vi "FPGA-test001.vi"() -> ()   [LabVIEW 2019]
uses:
  Labview/smallmom-3 FPGA test/FPGA-test/Sub VIs/Utilities/Start Boolean.ctl
  <vilib>/Platform/TimedLoop/XDataNode/timing_clust.ctl
  <vilib>/Platform/TimedLoop/XDataNode/nitl_modes.ctl
  <vilib>/Platform/TimedLoop/XDataNode/wakeup.ctl
  <vilib>/rvi/Emulation/niFpgaGetClockAttributes.vi
  <vilib>/rvi/Emulation/niFpgaSctlEmulationGetInTimedLoop.vi
  <vilib>/rvi/Emulation/niFpgaEmulationReportErrorSimple.vi
  <vilib>/rvi/eio/common/nirviEmuTemplateMethod_errors.vi
  <vilib>/rvi/Emulation/niFpgaCriticalErrorInLSC.vi
  <vilib>/eio/EIONode/EIONode.xnode
  <vilib>/platform/TimedLoop/XDataNode/XDataNode.xnode
  <vilib>/Platform/TimedLoop/XDataNode/XDNodeRunTimeDep.lvlib
panel:
  in  "Servo4.period (20Mhz)":u32=60606
  in  "Servo3.period (20Mhz)":u32=60606
  in  "Servo2.period (20Mhz)":u32=60606
  in  "Servo1.period (20Mhz)":u32=60606
  in  "Basic.2 IO Write":u8
  in  "Basic.2 IO DIR":u8
  out "Basic.2 IO Read":u8
  in  "Servo4.pulse(0.05us)":u32
  out "us4.distance":i32
  out "us3.distance":i32
  out "us2.distance":i32
  out "us1.distance":i32
  in  "us4.timeout(us)":i32
  in  "us3.timeout(us)":i32
  in  "us2.timeout(us)":i32
  in  "us1.timeout(us)":i32
  in  "Ultrasonic.IO.Enable":u8 format="%.0b"
  in  "I2C.A.GO":T1
  in  "I2C.A.CNFG":u8=1 format="%08b"
  out "I2C.A.STAT":u8 format="%08b"
  in  "I2C.A.CNTL":u8 format="%08b"
  in  "I2C.A.CNTR":u8=213
  in  "I2C.A.ADDR":u8 format="%08b"
  out "I2C.A.DATI":u8
  in  "I2C.A.DATO":u8
  in  "Ultrasonic.IO.Write":u8
  in  "Ultrasonic.io.DIR":u8
  out "Ultrasonic.io.Read":u8
  out "Basic IO Read":u8
  in  "Basic IO DIR":u8
  in  "Basic IO Write":u8
  out "IR 8":u16
  out "IR 7":u16
  out "IR 6":u16
  out "IR 5":u16
  out "IR 4":u16
  out "IR 3":u16
  out "IR 2":u16
  out "IR 1":u16
  in  "Servo3.pulse(0.05us)":u32
  in  "Servo2.pulse(0.05us)":u32
  in  "Servo1.pulse(0.05us)":u32
  in  "Motor3.encoder_Reset":bool
  out "Motor3.encoder":i32
  in  "Motor3.speed":i64
  in  "Motor3.periode":i64
  in  "Motor3.enable_divider":bool
  in  "Motor3.divider":fxp<+,4,4>
  in  "Motor3.brake":bool
  in  "Motor4.encoder_Reset":bool
  out "Motor4.encoder":i32
  in  "Motor4.speed":i64
  in  "Motor4.periode":i64
  in  "Motor4.enable_divider":bool
  in  "Motor4.divider":fxp<+,4,4>
  in  "Motor4.brake":bool
  in  "Motor2.encoder_Reset":bool
  out "Motor2.encoder":i32
  in  "Motor2.speed":i64
  in  "Motor2.periode":i64
  in  "Motor2.enable_divider":bool
  in  "Motor2.divider":fxp<+,4,4>
  in  "Motor2.brake":bool
  in  "Motor1.brake":bool
  in  "Motor1.divider":fxp<+,4,4>
  in  "Motor1.enable_divider":bool
  in  "Motor1.periode":i64
  in  "Motor1.speed":i64
  out "Motor1.encoder":i32
  in  "Motor1.encoder_Reset":bool
  out "OnBoard.BUTTON":bool
  in  "OnBoard.LED[3:0]":fxp<+,4,4> format="%.0b"
  # "Motor1"
  # "Motor2"
  # "Motor3"
  # "Motor4"
  # "Servo"
  # "IR Sensor"
  # "Basic IO"
  # "Ultrasonic IO"
  # "I2C"
  # "OnBoard"
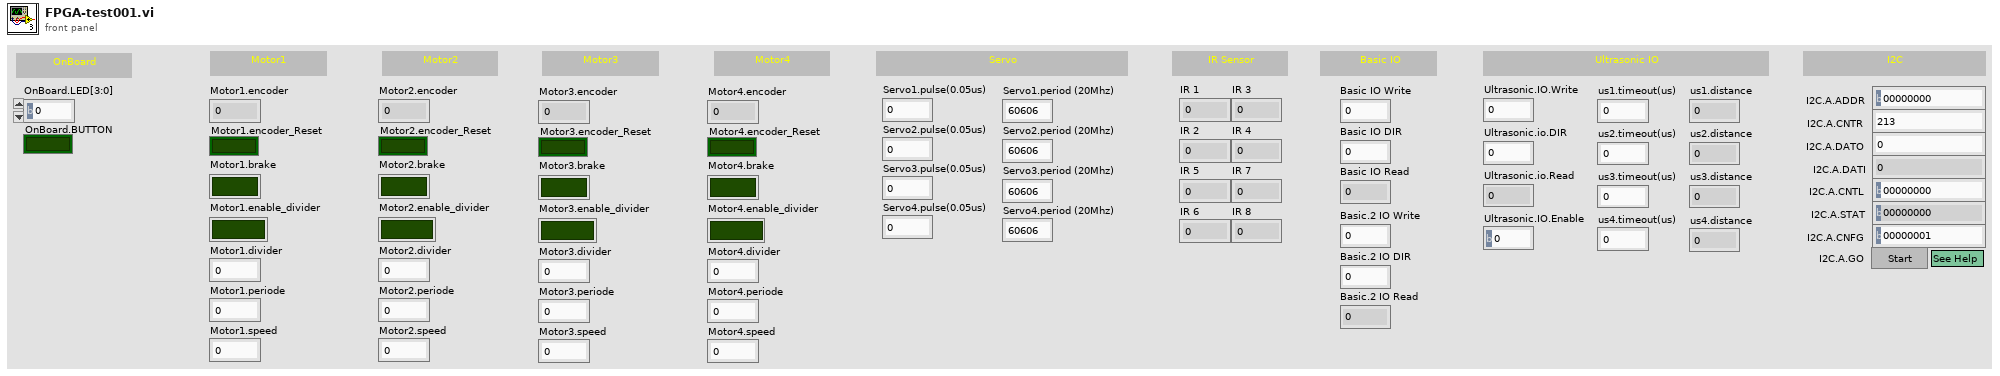
[diagram p1: front panel]
types:
  T1 = typedef "Start Boolean.ctl" = bool
  T2 = typedef "XDNodeRunTimeDep.lvlib/timing_clust.ctl" = cluster{"Expected End [f-1]":u64, "Actual End [f-1]":u64, "Finished Late? [f-1]":bool, "Expected End [i-1]":u64, "Actual End [i-1]":u64, "Finished Late? [i-1]":bool, "Expected Start [i]":u64, "Actual Start [i]":u64, "Expected Start [f]":u64, "Actual Start [f]":u64, "Source Name":string, "Structure Name":string, "Period":i64, "Deadline":i64, "Offset":i64, "Start":i64, "Priority":i32, "Timeout":i32, "Mode":T3, "Wakeup Reason":T4, "Error":errorcluster, "Source Type":string, "Secondary Source Type":string, "Global End Time":u64, "Global Start Time":u64, "Frame Duration":u64, "Iteration Duration":u64, "Assigned CPU":i32, "I/O Scan Engine Mode":u32}
  T3 = typedef "XDNodeRunTimeDep.lvlib/nitl_modes.ctl" = enum32{"No Change", "Process missed periods, maintain original phase", "Discard missed periods, maintain original phase", "Process missed periods, ignore original phase", "Discard missed periods, ignore original phase"}
  T4 = typedef "XDNodeRunTimeDep.lvlib/wakeup.ctl" = enum32{"Normal", "Aborted", "Asynchronous wakeup", "Timing source error", "Timed loop error", "Timeout"}
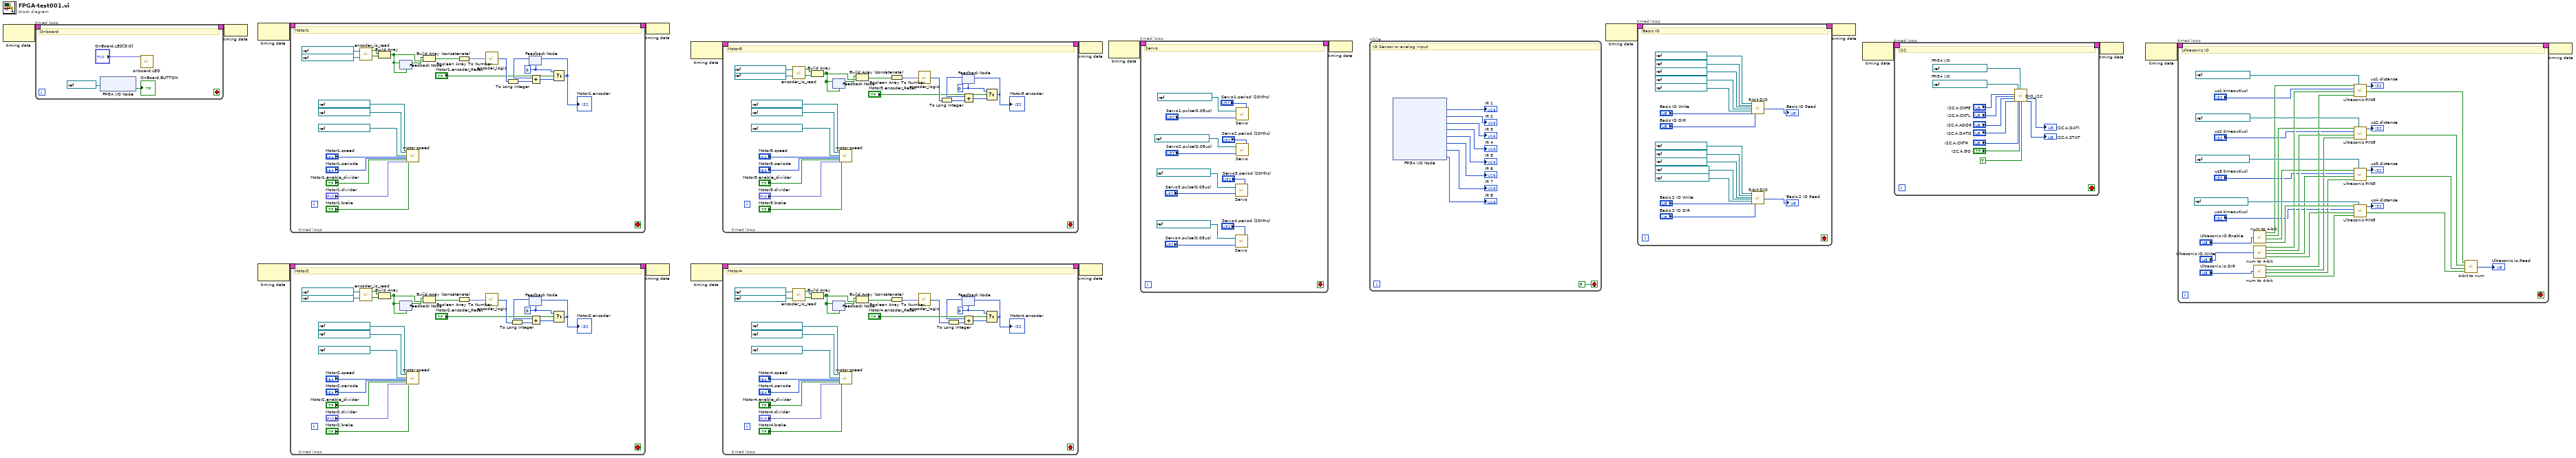
[diagram p0: block diagram]
diagram:
  n1 = node-c288() -> (w18:T2)  [unwired: 1 in]
  n2 = timed-loop "Timed Loop" {
    timing: w18 -> [_]
    timing-out: [_] -> w17
    stop <- _ stop-if-true
    # "Onboard"
    n3 = xnode "FPGA I/O Node"("FPGA I/O In"=refnum<k21> "Button0") -> ("I/O Item"=→"OnBoard.BUTTON":bool)  [unwired: 1 out]
    n4 = call "onboard.LED.vi"("OnBoard.LED[3:0]"="OnBoard.LED[3:0]") -> ()  [unwired: 11 in]
  }
  n5 = node-c288(w17) -> ()
  n6 = node-c288() -> (w16:T2)  [unwired: 1 in]
  n7 = node-c288() -> (w14:T2)  [unwired: 1 in]
  n8 = timed-loop "Timed Loop" {
    timing: w16 -> [_]
    timing-out: [_] -> w15
    stop <- _ stop-if-true
    w37 = 0
    # "Motor1"
    n9 = call "encoder_io_read.vi"("PhaseB"=refnum<k21> "ConnectorA/DIO3", "PhaseA"=refnum<k21> "ConnectorA/DIO2") -> ("PhaseB"=w44:bool, "PhaseA"=w45:bool)
    n10 = Build Array(w45, w44) -> (w42:bool[])
    n11 = feedback-in #1(w42) -> ()
    n12 = feedback #1(w42) -> (w43:bool[])
    n13 = call "motor speed.vi"("IN_A"=refnum<k21> "ConnectorA/DIO0" ("PhaseA"), "IN_B"=refnum<k21> "ConnectorA/DIO1" ("PhaseB"), "PWM"=refnum<k21> "ConnectorA/DIO4" ("PhaseB"), "speed"="Motor1.speed", "periode"="Motor1.periode", "enable divider"="Motor1.enable_divider", "divider"="Motor1.divider", "brake"="Motor1.brake") -> ()  [unwired: 20 in]
    n14 = Build Array (concatenate)(w43, w42) -> (w33:bool[])
    n15 = Boolean Array To Number(Boolean array=w33) -> (number=w41:fxp<+,4,4>)
    n16 = call "encoder_logic.vi"("encoder"=w41) -> ("out"=w39:i16)
    n17 = To Long Integer(number=w39) -> (32bit integer=w24:i32)
    n18 = feedback #2(w37) -> (w40:i32)
    n19 = Add(x=w40, y=w24) -> (x+y=w36:i32)
    n20 = Select(t=w37, s="Motor1.encoder_Reset", f=w36) -> (s? t:f=w35:i32)
    "Motor1.encoder" <- w35
    n21 = feedback-in #2(w35) -> ()
  }
  n22 = timed-loop "Timed Loop" {
    timing: w14 -> [_]
    timing-out: [_] -> w13
    stop <- _ stop-if-true
    w62 = 0
    # "Motor2"
    n23 = call "encoder_io_read.vi"("PhaseB"=refnum<k21> "ConnectorA/DIO8", "PhaseA"=refnum<k21> "ConnectorA/DIO7") -> ("PhaseB"=w69:bool, "PhaseA"=w70:bool)
    n24 = Build Array(w70, w69) -> (w67:bool[])
    n25 = feedback-in #3(w67) -> ()
    n26 = feedback #3(w67) -> (w68:bool[])
    n27 = call "motor speed.vi"("IN_A"=refnum<k21> "ConnectorA/DIO5" ("PhaseA"), "IN_B"=refnum<k21> "ConnectorA/DIO6" ("PhaseB"), "PWM"=refnum<k21> "ConnectorA/DIO9" ("PhaseB"), "speed"="Motor2.speed", "periode"="Motor2.periode", "enable divider"="Motor2.enable_divider", "divider"="Motor2.divider", "brake"="Motor2.brake") -> ()  [unwired: 20 in]
    n28 = Build Array (concatenate)(w68, w67) -> (w58:bool[])
    n29 = Boolean Array To Number(Boolean array=w58) -> (number=w66:fxp<+,4,4>)
    n30 = call "encoder_logic.vi"("encoder"=w66) -> ("out"=w64:i16)
    n31 = To Long Integer(number=w64) -> (32bit integer=w49:i32)
    n32 = feedback #4(w62) -> (w65:i32)
    n33 = Add(x=w65, y=w49) -> (x+y=w61:i32)
    n34 = Select(t=w62, s="Motor2.encoder_Reset", f=w61) -> (s? t:f=w60:i32)
    "Motor2.encoder" <- w60
    n35 = feedback-in #4(w60) -> ()
  }
  n36 = node-c288(w15) -> ()
  n37 = node-c288(w13) -> ()
  n38 = node-c288() -> (w12:T2)  [unwired: 1 in]
  n39 = node-c288() -> (w10:T2)  [unwired: 1 in]
  n40 = timed-loop "Timed Loop" {
    timing: w12 -> [_]
    timing-out: [_] -> w11
    stop <- _ stop-if-true
    w87 = 0
    # "Motor3"
    n41 = call "encoder_io_read.vi"("PhaseB"=refnum<k21> "ConnectorB/DIO3", "PhaseA"=refnum<k21> "ConnectorB/DIO2") -> ("PhaseB"=w94:bool, "PhaseA"=w95:bool)
    n42 = Build Array(w95, w94) -> (w92:bool[])
    n43 = feedback-in #5(w92) -> ()
    n44 = feedback #5(w92) -> (w93:bool[])
    n45 = call "motor speed.vi"("IN_A"=refnum<k21> "ConnectorB/DIO0" ("PhaseA"), "IN_B"=refnum<k21> "ConnectorB/DIO1" ("PhaseB"), "PWM"=refnum<k21> "ConnectorB/DIO4" ("PhaseB"), "speed"="Motor3.speed", "periode"="Motor3.periode", "enable divider"="Motor3.enable_divider", "divider"="Motor3.divider", "brake"="Motor3.brake") -> ()  [unwired: 20 in]
    n46 = Build Array (concatenate)(w93, w92) -> (w83:bool[])
    n47 = Boolean Array To Number(Boolean array=w83) -> (number=w91:fxp<+,4,4>)
    n48 = call "encoder_logic.vi"("encoder"=w91) -> ("out"=w89:i16)
    n49 = To Long Integer(number=w89) -> (32bit integer=w74:i32)
    n50 = feedback #6(w87) -> (w90:i32)
    n51 = Add(x=w90, y=w74) -> (x+y=w86:i32)
    n52 = Select(t=w87, s="Motor3.encoder_Reset", f=w86) -> (s? t:f=w85:i32)
    "Motor3.encoder" <- w85
    n53 = feedback-in #6(w85) -> ()
  }
  n54 = timed-loop "Timed Loop" {
    timing: w10 -> [_]
    timing-out: [_] -> w9
    stop <- _ stop-if-true
    w112 = 0
    # "Motor4"
    n55 = call "encoder_io_read.vi"("PhaseB"=refnum<k21> "ConnectorB/DIO8", "PhaseA"=refnum<k21> "ConnectorB/DIO7") -> ("PhaseB"=w119:bool, "PhaseA"=w120:bool)
    n56 = Build Array(w120, w119) -> (w117:bool[])
    n57 = feedback-in #7(w117) -> ()
    n58 = feedback #7(w117) -> (w118:bool[])
    n59 = call "motor speed.vi"("IN_A"=refnum<k21> "ConnectorB/DIO5" ("PhaseA"), "IN_B"=refnum<k21> "ConnectorB/DIO6" ("PhaseB"), "PWM"=refnum<k21> "ConnectorB/DIO9" ("PhaseB"), "speed"="Motor4.speed", "periode"="Motor4.periode", "enable divider"="Motor4.enable_divider", "divider"="Motor4.divider", "brake"="Motor4.brake") -> ()  [unwired: 20 in]
    n60 = Build Array (concatenate)(w118, w117) -> (w108:bool[])
    n61 = Boolean Array To Number(Boolean array=w108) -> (number=w116:fxp<+,4,4>)
    n62 = call "encoder_logic.vi"("encoder"=w116) -> ("out"=w114:i16)
    n63 = To Long Integer(number=w114) -> (32bit integer=w99:i32)
    n64 = feedback #8(w112) -> (w115:i32)
    n65 = Add(x=w115, y=w99) -> (x+y=w111:i32)
    n66 = Select(t=w112, s="Motor4.encoder_Reset", f=w111) -> (s? t:f=w110:i32)
    "Motor4.encoder" <- w110
    n67 = feedback-in #8(w110) -> ()
  }
  n68 = node-c288(w11) -> ()
  n69 = node-c288(w9) -> ()
  n70 = node-c288() -> (w8:T2)  [unwired: 1 in]
  n71 = timed-loop {
    timing: w8 -> [_]
    timing-out: [_] -> w7
    stop <- _ stop-if-true
    # "Servo"
    n72 = call "Servo.vi"("period (20Mhz)"="Servo3.period (20Mhz)", "(2.5us)"="Servo3.pulse(0.05us)", "Servo DIO"=refnum<k21> "ConnectorB/DIO10") -> ()
    n73 = call "Servo.vi"("period (20Mhz)"="Servo4.period (20Mhz)", "(2.5us)"="Servo4.pulse(0.05us)", "Servo DIO"=refnum<k21> "ConnectorB/DIO11") -> ()
    n74 = call "Servo.vi"("period (20Mhz)"="Servo1.period (20Mhz)", "(2.5us)"="Servo1.pulse(0.05us)", "Servo DIO"=refnum<k21> "ConnectorA/DIO10") -> ()
    n75 = call "Servo.vi"("period (20Mhz)"="Servo2.period (20Mhz)", "(2.5us)"="Servo2.pulse(0.05us)", "Servo DIO"=refnum<k21> "ConnectorA/DIO11") -> ()
  }
  n76 = node-c288(w7) -> ()
  n77 = while {
    stop <- FALSE stop-if-true
    # "IR Sensor or analog input"
    n78 = xnode "FPGA I/O Node"() -> ("ConnectorA/AI0"=→"IR 1":u16, "ConnectorA/AI1"=→"IR 2":u16, "ConnectorA/AI2"=→"IR 3":u16, "ConnectorA/AI3"=→"IR 4":u16, "ConnectorB/AI0"=→"IR 5":u16, "ConnectorB/AI1"=→"IR 6":u16, "ConnectorB/AI2"=→"IR 7":u16, "ConnectorB/AI3"=→"IR 8":u16)  [unwired: 8 in, 8 out]
  }
  n79 = node-c288() -> (w6:T2)  [unwired: 1 in]
  n80 = timed-loop {
    timing: w6 -> [_]
    timing-out: [_] -> w5
    stop <- _ stop-if-true
    # "Basic IO"
    n81 = call "5-bit DIO.vi"("DIO Refnum 1"=refnum<k21> "ConnectorC/DIO0", "DIO Refnum 2"=refnum<k21> "ConnectorC/DIO1" ("DIO Refnum 1"), "DIO Refnum 3"=refnum<k21> "ConnectorC/DIO2" ("DIO Refnum 1"), "DIO Refnum 4"=refnum<k21> "ConnectorC/DIO3" ("DIO Refnum 1"), "DIO Refnum 5"=refnum<k21> "ConnectorC/DIO4" ("DIO Refnum 1"), "DIO OUT[4:0]"="Basic IO Write", "DIO DIR[4:0]"="Basic IO DIR") -> ("DIO IN[4:0]"=→"Basic IO Read":u8)  [unwired: 12 in]
    n82 = call "5-bit DIO.vi"("DIO Refnum 1"=refnum<k21> "ConnectorC/DIO5", "DIO Refnum 2"=refnum<k21> "ConnectorC/DIO6" ("DIO Refnum 1"), "DIO Refnum 3"=refnum<k21> "ConnectorC/DIO7" ("DIO Refnum 1"), "DIO Refnum 4"=refnum<k21> "ConnectorB/DIO14" ("DIO Refnum 1"), "DIO Refnum 5"=refnum<k21> "ConnectorB/DIO15" ("DIO Refnum 1"), "DIO OUT[4:0]"="Basic.2 IO Write", "DIO DIR[4:0]"="Basic.2 IO DIR") -> ("DIO IN[4:0]"=→"Basic.2 IO Read":u8)  [unwired: 12 in]
  }
  n83 = node-c288(w5) -> ()
  n84 = node-c288() -> (w2:T2)  [unwired: 1 in]
  n85 = timed-loop {
    timing: w2 -> [_]
    timing-out: [_] -> w1
    stop <- _ stop-if-true
    w166 = refnum<k21> "ConnectorA/DIO15"  # FPGA I/O
    w167 = refnum<k21> "ConnectorA/DIO14"  # FPGA I/O
    # "I2C"
    n86 = call "DIO_I2C.vi"("I2C.CNFG"="I2C.A.CNFG", "I2C.CNTL"="I2C.A.CNTL", "I2C.ADDR"="I2C.A.ADDR", "I2C.DATO"="I2C.A.DATO", "DIO.1/I2C.SDA"=w166, "I2C.CNTR"="I2C.A.CNTR", "DIO.0/I2C.SCL"=w167, "Execute?"="I2C.A.GO", "SELECT"=TRUE) -> ("I2C.DATI"=→"I2C.A.DATI":u8, "I2C.STAT"=→"I2C.A.STAT":u8)  [unwired: 8 in, 1 out]
  }
  n87 = node-c288(w1) -> ()
  n88 = node-c288() -> (w4:T2)  [unwired: 1 in]
  n89 = timed-loop {
    timing: w4 -> [_]
    timing-out: [_] -> w3
    stop <- _ stop-if-true
    # "Ultrasonic IO"
    n90 = call "num to 4-bit.vi"("DIO DIR[3:0]"="Ultrasonic.IO.Enable") -> ("element"=w202:bool, "element 2"=w201:bool, "element 3"=w200:bool, "element 4"=w199:bool)
    n91 = call "num to 4-bit.vi"("DIO DIR[3:0]"="Ultrasonic.IO.Write") -> ("element"=w198:bool, "element 2"=w197:bool, "element 3"=w196:bool, "element 4"=w195:bool)
    n92 = call "num to 4-bit.vi"("DIO DIR[3:0]"="Ultrasonic.io.DIR") -> ("element"=w194:bool, "element 2"=w193:bool, "element 3"=w192:bool, "element 4"=w191:bool)
    n93 = call "ultrasonic PING.vi"("DIO Refnum"=refnum<k21> "ConnectorA/DIO12" ("DIO Refnum 1"), "DIR"=w194, "OUT"=w198, "timeout(us)"="us1.timeout(us)", "F selection"=w202) -> ("IN"=w189:bool, "ultrasonic output"=→"us1.distance":i32)  [unwired: 5 in]
    n94 = call "ultrasonic PING.vi"("DIO Refnum"=refnum<k21> "ConnectorA/DIO13" ("DIO Refnum 1"), "DIR"=w193, "OUT"=w197, "timeout(us)"="us2.timeout(us)", "F selection"=w201) -> ("IN"=w188:bool, "ultrasonic output"=→"us2.distance":i32)  [unwired: 5 in]
    n95 = call "ultrasonic PING.vi"("DIO Refnum"=refnum<k21> "ConnectorB/DIO12" ("DIO Refnum 1"), "DIR"=w192, "OUT"=w196, "timeout(us)"="us3.timeout(us)", "F selection"=w200) -> ("IN"=w187:bool, "ultrasonic output"=→"us3.distance":i32)  [unwired: 5 in]
    n96 = call "ultrasonic PING.vi"("DIO Refnum"=refnum<k21> "ConnectorB/DIO13" ("DIO Refnum 1"), "DIR"=w191, "OUT"=w195, "timeout(us)"="us4.timeout(us)", "F selection"=w199) -> ("IN"=w186:bool, "ultrasonic output"=→"us4.distance":i32)  [unwired: 5 in]
    n97 = call "4-bit to num.vi"("Boolean 4"=w186, "Boolean 3"=w187, "Boolean 2"=w188, "Boolean"=w189) -> ("DIO IN[3:0]"=→"Ultrasonic.io.Read":u8)
  }
  n98 = node-c288(w3) -> ()
